vi "_Generate_Dictionary_for_VI.vi"() -> ()   [LabVIEW 2019]
uses:
  <userlib>/_OpenG.lib/array/array.llb/Remove Duplicates from 1D Array (String)__ogtk.vi
  <userlib>/_OpenG.lib/array/array.llb/Delete Elements from 2D Array (String)__ogtk.vi
panel:
  out "dictionary_save_path":path caption="selected path"
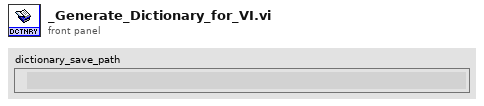
[diagram p1: front panel]
types:
  T1 = enum16{"open", "replace", "create", "open or create", "replace or create", "replace or create with confirmation"}
  T2 = enum32{"invalid OS target", "Mac OS", "Windows 3.1", "Windows 95/NT", "Solaris 1", "Solaris 2", "HP-UX", "PowerMAX", "Linux", "Irix", "Rhapsody", "BeOS", "AIX", "OSF1", "VxWorks", "PharLap", "Carbon", "RTX", "Windows x64", "Linux x64", "Mac OS X x64"}
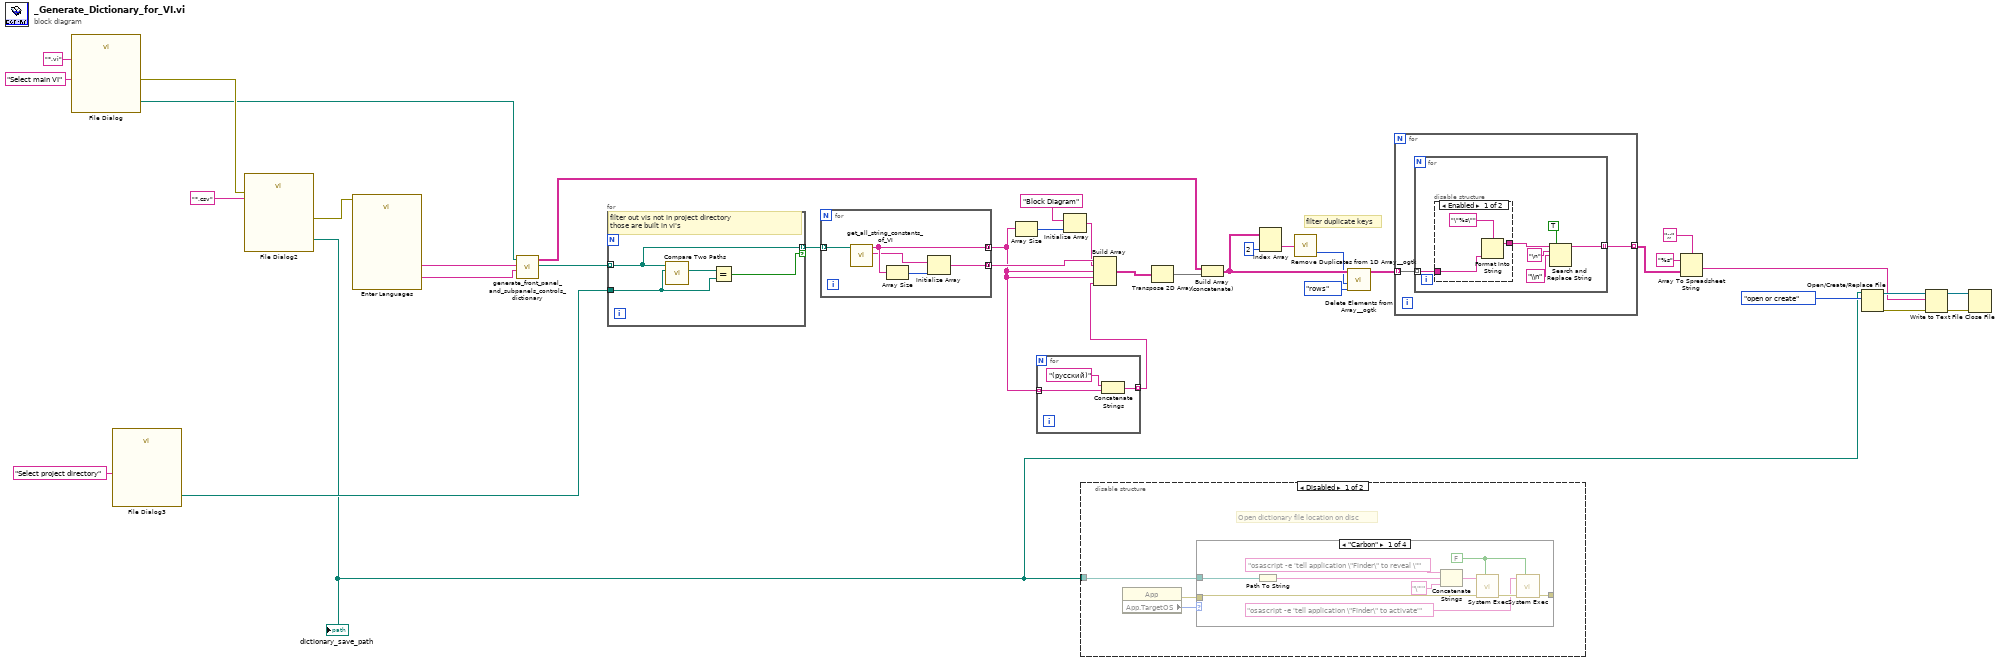
[diagram p0: block diagram]
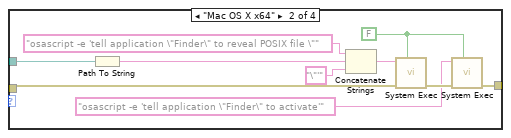
[diagram p3: hidden frame]
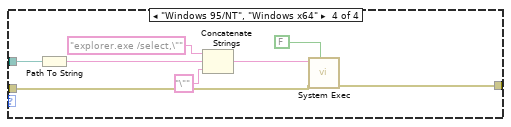
[diagram p5: hidden frame]
diagram:
  # "filter duplicate keys"
  n1 = call "File Dialog"("prompt"="Select main VI", "pattern (all files)"="*.vi" ("pattern label")) -> ("selected path"=w33:path, "error out"=w35:errorcluster)  [unwired: 10 in, 2 out]
  n2 = call "File Dialog3"("prompt"="Select project directory") -> ("selected path"=w29:path)  [unwired: 11 in, 3 out]
  n3 = call "File Dialog2"("error in"=w35, "pattern (all files)"="*.csv" ("pattern label")) -> ("selected path"=w7:path, "error out"=w34:errorcluster)  [unwired: 10 in, 2 out]
  "dictionary_save_path" <- w7
  n4 = call "Enter Languages"("error in (no error)"=w34) -> ("Additional Language"=w31:string, "Current Language"=w32:string)  [unwired: 15 in, 2 out]
  n5 = call "generate_front_panel_and_subpanels_controls_dictionary.vi"("additional_language"=w31, "current_language"=w32, "main_VI_path"=w33) -> ("all_paths"=w27:path[], "panels_dictionary_array"=w23:string[][])  [unwired: 7 in]
  n6 = for {
    tunnel: w27 -> [w41] mode=indexing
    tunnel: w29 -> [w39]
    tunnel: [w41] -> w26 mode=indexing if=w38
    # "filter out vis not in project directory\nthose are built in vi's"
    n7 = call <vilib>:"Compare Two Paths.vi"("Path 2"=w39, "Path 1"=w41) -> ("Common Path"=w40:path)  [unwired: 6 in, 3 out]
    n8 = Equal?(x=w40, y=w39) -> (x = y?=w38:bool)
  }
  n9 = for {
    tunnel: [w45] -> w2 mode=concatenating
    tunnel: w26 -> [w46] mode=indexing
    tunnel: [w42] -> w4 mode=concatenating
    n10 = call "get_all_string_constants_of_VI.vi"("VI_path"=w46) -> ("VI_name"=w43:string, "string_constants"=w45:string[])  [unwired: 9 in]
    n11 = Array Size(array=w45) -> (size(s)=w44:i32)
    n12 = Initialize Array(w43, w44) -> (w42:string[])
  }
  n13 = Array Size(array=w2) -> (size(s)=w17:i32)
  n14 = for {
    tunnel: w2 -> [w48] mode=indexing
    tunnel: [w47] -> w1 mode=indexing
    n15 = Concatenate Strings("(русский)", w48) -> (w47:string)
  }
  n16 = Initialize Array("Block Diagram" ("element"), w17) -> (w3:string[])
  n17 = disable-structure shown="Disabled" {
    disable-tunnel: w7 -> [w50 _]
    frame Disabled {
      # "Open dictionary file location on disc"
      n18 = property class="App"() -> (error out=w51:errorcluster, "App.TargetOS"=w52:T2)  [unwired: 2 in, 1 out]
      n19 = case shown="\"Carbon\"" w52 {
        tunnel: w50 -> [w55 w67 _ w77]
        tunnel: w51 -> [w53 w63 w73 w75]
        tunnel: [w54 w64 w73 w74] -> _
        frame "Carbon" {
          w58 = FALSE ("wait until completion? (T)")
          n20 = Path To String(path=w55) -> (string=w56:string)
          n21 = Concatenate Strings("osascript -e 'tell application \"Finder\" to reveal \"" ("string"), w56, "\"'" ("string")) -> (w60:string)
          n22 = call <vilib>:"System Exec.vi"("wait until completion? (T)"=w58, "error in (no error)"=w53, "command line"=w60) -> ("error out"=w59:errorcluster)  [unwired: 5 in, 3 out]
          n23 = call <vilib>:"System Exec.vi"("wait until completion? (T)"=w58, "error in (no error)"=w59, "command line"="osascript -e 'tell application \"Finder\" to activate'" ("string")) -> ("error out"=w54:errorcluster)  [unwired: 5 in, 3 out]
        }
        frame "Mac OS X x64" {
          w69 = FALSE ("wait until completion? (T)")
          n24 = Path To String(path=w67) -> (string=w66:string)
          n25 = Concatenate Strings("osascript -e 'tell application \"Finder\" to reveal POSIX file \"" ("string"), w66, "\"'" ("string")) -> (w71:string)
          n26 = call <vilib>:"System Exec.vi"("wait until completion? (T)"=w69, "error in (no error)"=w63, "command line"=w71) -> ("error out"=w70:errorcluster)  [unwired: 5 in, 3 out]
          n27 = call <vilib>:"System Exec.vi"("wait until completion? (T)"=w69, "error in (no error)"=w70, "command line"="osascript -e 'tell application \"Finder\" to activate'" ("string")) -> ("error out"=w64:errorcluster)  [unwired: 5 in, 3 out]
        }
        frame Default {
        }
        frame "Windows 95/NT", "Windows x64" {
          n28 = Path To String(path=w77) -> (string=w76:string)
          n29 = Concatenate Strings("explorer.exe /select,\"" ("string"), w76, "\"" ("string")) -> (w79:string)
          n30 = call <vilib>:"System Exec.vi"("wait until completion? (T)"=FALSE, "error in (no error)"=w75, "command line"=w79) -> ("error out"=w74:errorcluster)  [unwired: 5 in, 3 out]
        }
      }
    }
    frame Enabled {
    }
  }
  n31 = Build Array(w4, w3, w2, w2, w1) -> (w25:string[][])
  n32 = Transpose 2D Array(2D array=w25) -> (transposed array=w24:string[][])
  n33 = Build Array (concatenate)(w23, w24) -> (w20:string[][])
  n34 = Index Array(array=w20, index (col)=2 ("disabled index (col)")) -> (element=w21:string[])  [unwired: 1 in]
  n35 = call-poly <userlib>:"Remove Duplicates from 1D Array__ogtk.vi"("Input Array"=w21) -> ("indices of removed elements"=w19:i32[])  [unwired: 1 out]
  n36 = call-poly <userlib>:"Delete Elements from Array__ogtk.vi"("delete (rows or columns)"=enum16{"rows", "columns"}."rows", "indices"=w19, "array"=w20) -> ("array w/ subset deleted"=w6:string[][])  [unwired: 7 in, 1 out]
  n37 = for {
    tunnel: w6 -> [w83] mode=indexing
    tunnel: [w82] -> w5 mode=indexing
    n38 = for {
      tunnel: w83 -> [w89] mode=indexing
      tunnel: [w86] -> w82 mode=indexing
      n39 = disable-structure shown="Enabled" {
        disable-tunnel: w89 -> [w92 w93]
        disable-tunnel: [w90 w93] -> w88
        frame Enabled {
          n40 = Format Into String(format string="\"%s\"", w92) -> (resulting string=w90:string)  [unwired: 2 in, 1 out]
        }
        frame Disabled {
        }
      }
      n41 = Search and Replace String(replace all?=TRUE ("replace all? (F)"), input string=w88, search string="\n", replace string="\\n" ("replace string (\"\")")) -> (result string=w86:string)  [unwired: 4 in, 3 out]
    }
  }
  n42 = Array To Spreadsheet String(delimiter (Tab)=";;", array=w5, 3:"%s" ("format string")) -> (spreadsheet string=w8:string)
  n43 = Open/Create/Replace File(file path (use dialog)=w7, operation (0:open)=T1."open or create") -> (refnum out=w10:refnum<file>, error out=w9:errorcluster)  [unwired: 4 in, 1 out]
  n44 = Write to Text File(file (use dialog)=w10, text=w8, error in=w9) -> (refnum out=w11:refnum<file>, error out=w12:errorcluster)  [unwired: 1 in, 1 out]
  n45 = Close File(refnum=w11, error in=w12) -> ()  [unwired: 2 out]
